vi "Matrix left division.vi"   [LabVIEW 2020, in "NI_Gmath.lvlib"]
uses:
  <vilib>/gmath/NI_Gmath.lvlib
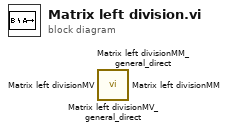
[diagram p0: block diagram]
diagram:
  n1 = call <vilib>:"Matrix left divisionMV_general_direct.vi"() -> ()  [unwired: 4 in, 2 out]
  n2 = call <vilib>:"Matrix left divisionMM_general_direct.vi"() -> ()  [unwired: 4 in, 2 out]
  n3 = call <vilib>:"Matrix left divisionMV.vi"() -> ()  [unwired: 4 in, 2 out]
  n4 = call <vilib>:"Matrix left divisionMM.vi"() -> ()  [unwired: 4 in, 2 out]
